vi "add_xml_file_headers.vi"(10 "xml":string) -> (3 "xml with headers":string)   [LabVIEW 2013]
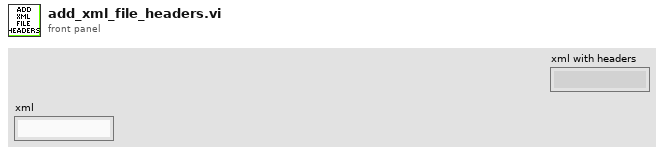
[diagram p1: front panel]
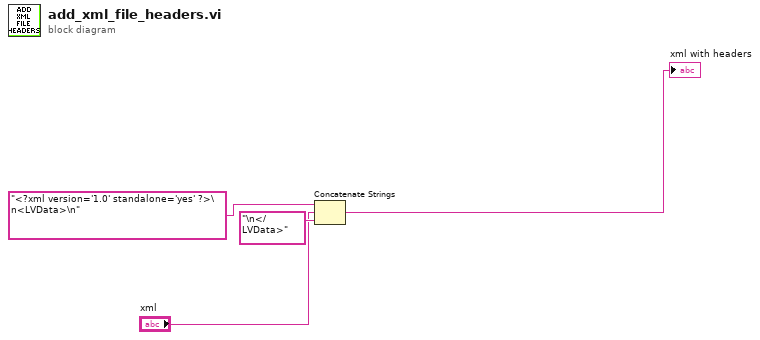
[diagram p0: block diagram]
diagram:
  n1 = Concatenate Strings("<?xml version='1.0' standalone='yes' ?>\n<LVData>\n", "xml", "\n</LVData>" ("string")) -> (→"xml with headers":string)
